vi "Cal(SubVI)-2013.vi"(0 "Array":dbl[][](array[numeric]), 1 "dt":sgl, 2 "StartChan":i32=32, 3 "tstart":sgl, 5 "FitData":dbl[][](array[numeric])) -> (6 "plot(Signals) 1-32":T2, 10 "plot(Signals) 33-64":T1)   [LabVIEW 2014]
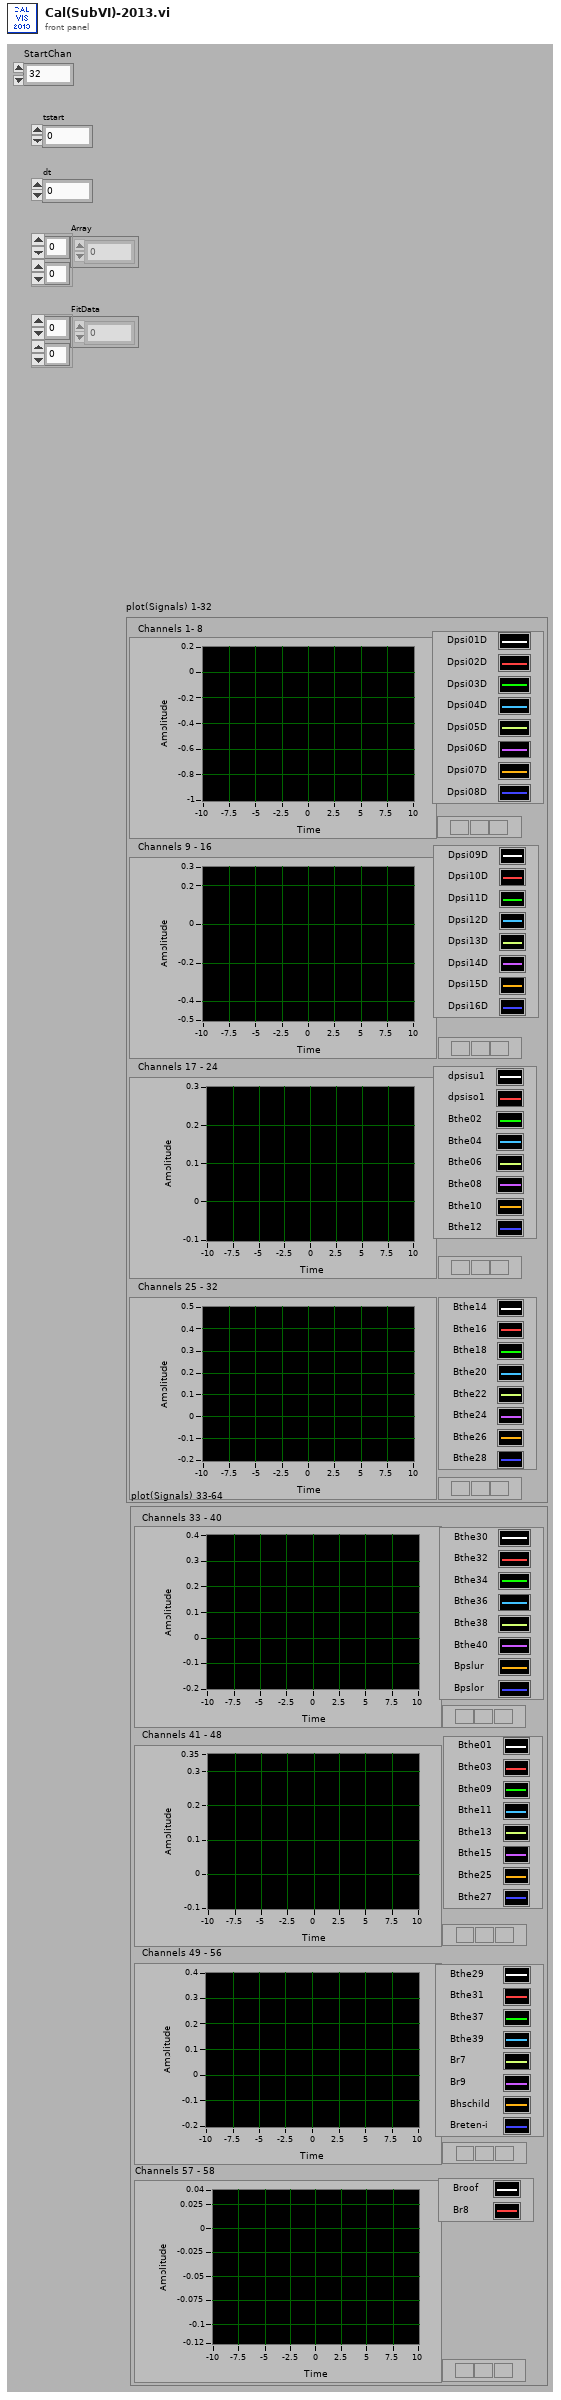
[diagram p1: front panel]
types:
  T1 = cluster{"Channels 33 - 40":cluster{"tstart":sgl, "dt":sgl, "OutArray":dbl[][]}, "Channels 41 - 48":cluster{"tstart":sgl, "dt":sgl, "OutArray":dbl[][]}, "Channels 49 - 56":cluster{"tstart":sgl, "dt":sgl, "OutArray":dbl[][]}, "Channels 57 - 58":cluster{"tstart":sgl, "dt":sgl, "OutArray":dbl[][]}}
  T2 = cluster{"Channels 1- 8":cluster{"tstart":sgl, "dt":sgl, "OutArray":dbl[][]}, "Channels 9 - 16":cluster{"tstart":sgl, "dt":sgl, "OutArray":dbl[][]}, "Channels 17 - 24":cluster{"tstart":sgl, "dt":sgl, "OutArray":dbl[][]}, "Channels 25 - 32":cluster{"tstart":sgl, "dt":sgl, "OutArray":dbl[][]}}
  T3 = cluster{"tstart":sgl, "dt":sgl, "OutArray":dbl[][]}
  T4 = cluster{cluster{"tstart":sgl, "dt":sgl, "OutArray":dbl[][]}, cluster{"tstart":sgl, "dt":sgl, "OutArray":dbl[][]}, cluster{"tstart":sgl, "dt":sgl, "OutArray":dbl[][]}, cluster{"tstart":sgl, "dt":sgl, "OutArray":dbl[][]}}
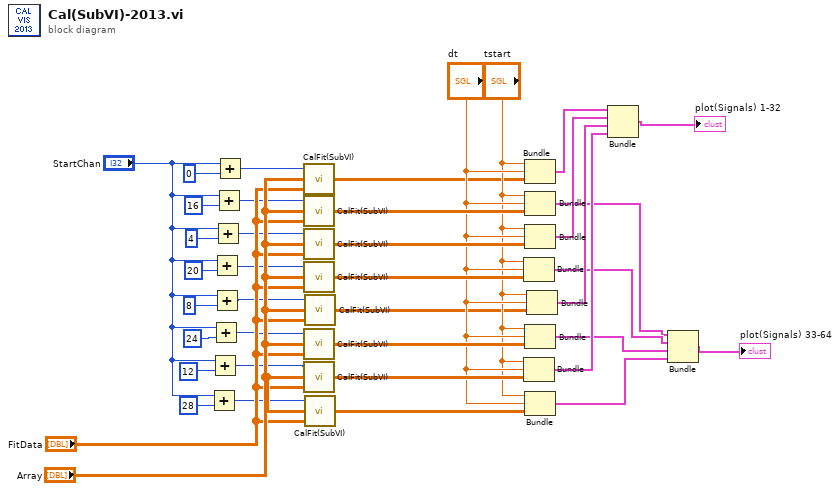
[diagram p0: block diagram]
diagram:
  n1 = Add(x="StartChan", y=28) -> (x+y=w12:i32)
  n2 = Add(x="StartChan", y=12) -> (x+y=w14:i32)
  n3 = Add(x="StartChan", y=24) -> (x+y=w16:i32)
  n4 = Add(x="StartChan", y=20) -> (x+y=w20:i32)
  n5 = Add(x="StartChan", y=8) -> (x+y=w18:i32)
  n6 = Add(x="StartChan", y=4) -> (x+y=w22:i32)
  n7 = Add(x="StartChan", y=16) -> (x+y=w24:i32)
  n8 = Add(x="StartChan", y=0) -> (x+y=w26:i32)
  n9 = call "CalFit(SubVI).vi"("FitData"="FitData", "Calcurrent"="Array", "Index"=w26) -> ("OutArray"=w28:dbl[][])
  n10 = call "CalFit(SubVI).vi"("FitData"="FitData", "Calcurrent"="Array", "Index"=w24) -> ("OutArray"=w35:dbl[][])
  n11 = call "CalFit(SubVI).vi"("FitData"="FitData", "Calcurrent"="Array", "Index"=w22) -> ("OutArray"=w36:dbl[][])
  n12 = call "CalFit(SubVI).vi"("FitData"="FitData", "Calcurrent"="Array", "Index"=w20) -> ("OutArray"=w34:dbl[][])
  n13 = call "CalFit(SubVI).vi"("FitData"="FitData", "Calcurrent"="Array", "Index"=w16) -> ("OutArray"=w32:dbl[][])
  n14 = call "CalFit(SubVI).vi"("FitData"="FitData", "Calcurrent"="Array", "Index"=w14) -> ("OutArray"=w37:dbl[][])
  n15 = call "CalFit(SubVI).vi"("FitData"="FitData", "Calcurrent"="Array", "Index"=w18) -> ("OutArray"=w29:dbl[][])
  n16 = call "CalFit(SubVI).vi"("FitData"="FitData", "Calcurrent"="Array", "Index"=w12) -> ("OutArray"=w33:dbl[][])
  n17 = Bundle("tstart"="tstart", "dt"="dt", "OutArray"=w34) -> (w3:T3)  [unwired: 1 out]
  n18 = Bundle("tstart"="tstart", "dt"="dt", "OutArray"=w37) -> (w7:T3)  [unwired: 1 out]
  n19 = Bundle("tstart"="tstart", "dt"="dt", "OutArray"=w28) -> (w10:T3)  [unwired: 1 out]
  n20 = Bundle("tstart"="tstart", "dt"="dt", "OutArray"=w35) -> (w2:T3)  [unwired: 1 out]
  n21 = Bundle("tstart"="tstart", "dt"="dt", "OutArray"=w36) -> (w9:T3)  [unwired: 1 out]
  n22 = Bundle("tstart"="tstart", "dt"="dt", "OutArray"=w32) -> (w4:T3)  [unwired: 1 out]
  n23 = Bundle("tstart"="tstart", "dt"="dt", "OutArray"=w33) -> (w5:T3)  [unwired: 1 out]
  n24 = Bundle("tstart"="tstart", "dt"="dt", "OutArray"=w29) -> (w8:T3)  [unwired: 1 out]
  n25 = Bundle(w10, w9, w8, w7) -> (→"plot(Signals) 1-32":T4)  [unwired: 1 out]
  n26 = Bundle(w2, w3, w4, w5) -> (→"plot(Signals) 33-64":T4)  [unwired: 1 out]
